vi "Set Row Height.vi"(8 "error in":errorcluster, 9 "Height":i32, 10 "Row":i32, 11 "SourceGrid in":refnum<class "SourceGrid.lvclass">) -> (0 "error out":errorcluster, 3 "SourceGrid out":refnum<class "SourceGrid.lvclass">)   [LabVIEW 2024, in "SourceGrid.lvlib" / "SourceGrid.lvclass"]
uses:
  SourceGrid.lvclass
  SourceGrid.lvclass/SourceGrid.ctl
  D:/git/Sourcegrid-LabVIEW/dll/SourceGrid.dll
  dll/SourceGrid.dll
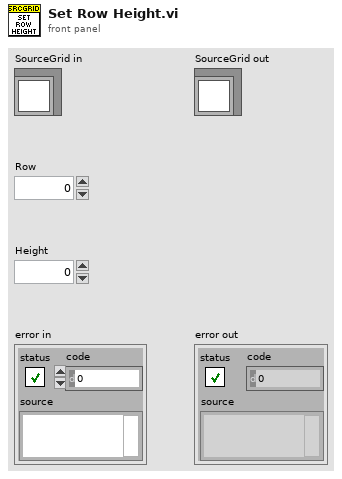
[diagram p1: front panel]
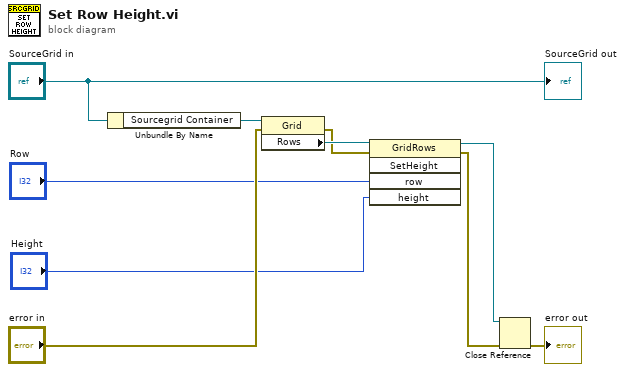
[diagram p0: block diagram]
diagram:
  n1 = Unbundle By Name("SourceGrid in") -> ("Sourcegrid Container"=w9:refnum<k24>)
  n2 = property class="Grid"(reference=w9, error in="error in") -> (error out=w4:errorcluster, "Rows"=w7:refnum<k24>)  [unwired: 1 out]
  n3 = invoke class="GridRows" method="SetHeight"(reference=w7, error in=w4, "row"="Row", "height"="Height") -> (reference out=w1:refnum<k24>, error out=w3:errorcluster)  [unwired: 1 in, 3 out]
  n4 = Close Reference(reference=w1, error in (no error)=w3) -> (error out=→"error out":errorcluster)
  "SourceGrid out" <- "SourceGrid in"
